vi "Start Recording.vi"(8 "error in (no error)":errorcluster, 10 "Update rate":dbl, 11 "Red Pitaya in":refnum<class "Red Pitaya.lvclass">) -> (0 "error out":errorcluster, 3 "Red Pitaya out":refnum<class "Red Pitaya.lvclass">)   [LabVIEW 2015]
uses:
  Red Pitaya.lvclass
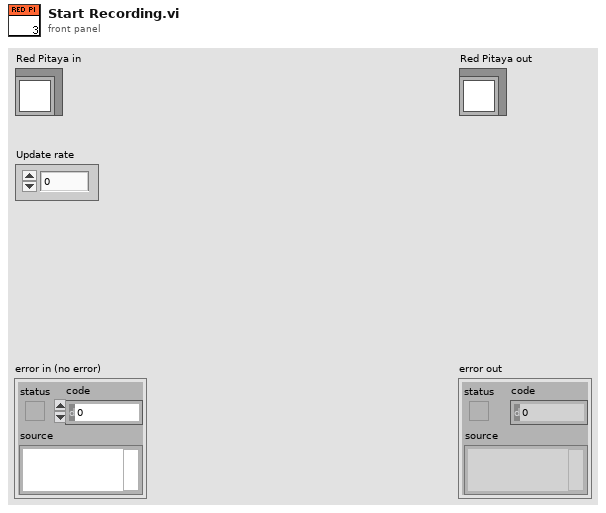
[diagram p1: front panel]
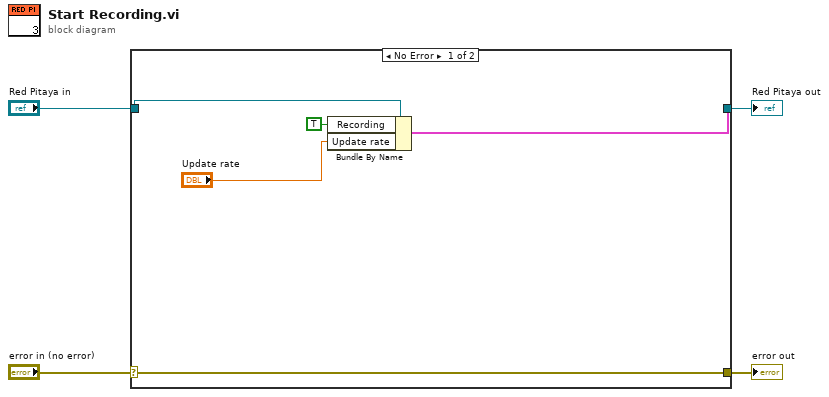
[diagram p0: block diagram]
diagram:
  n1 = case shown="No Error" "error in (no error)" {
    selector: "error in (no error)" -> [w8 w11]
    tunnel: [w8 w11] -> w3
    tunnel: [w7 w10] -> w1
    tunnel: "Red Pitaya in" -> [w9 w10]
    frame No Error {
      n2 = Bundle By Name(cluster=w9, "Recording"=TRUE, "Update rate"="Update rate") -> (w7:cluster{})
    }
    frame Error {
    }
  }
  "error out" <- w3
  "Red Pitaya out" <- w1
